vi "KundtsTube.vi"() -> ()   [LabVIEW 2014]
panel:
  in  "Amplitude":dbl
  in  "Stop":bool
  in  "?":enum32{"Sweep", "Single"}(tab)
  in  "Dwell Time":dbl
  in  "Frequency":dbl
  in  "Input 2":T1
  out "RMS":dbl
  out "Waveform Graph":dynamicdata(graph)
  in  "Input":T2
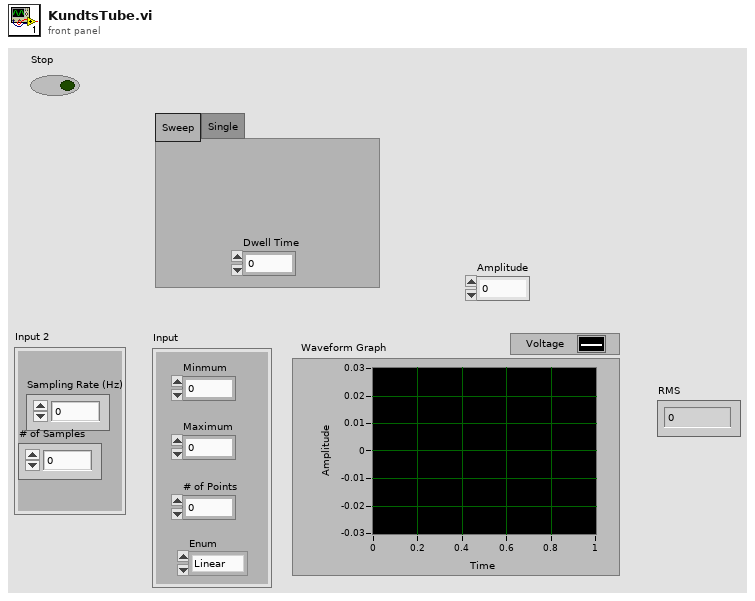
[diagram p1: front panel]
types:
  T1 = cluster{"Sampling Rate (Hz)":dbl, "# of Samples":i64}
  T2 = cluster{"Minmum":i64, "Maximum":i64, "# of Points":i64, "Enum":enum16{"Linear", "Logarithmic", ""}}
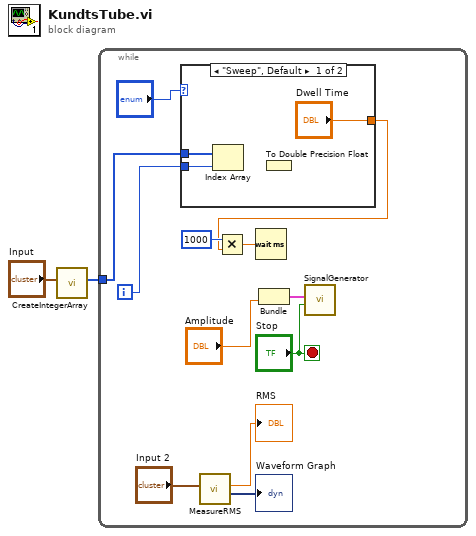
[diagram p0: block diagram]
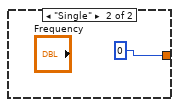
[diagram p2: hidden frame]
diagram:
  n1 = call "CreateIntegerArray.vi"("Input"="Input") -> ("Output Array"=w1:i64[])  [unwired: 10 in]
  n2 = while {
    tunnel: w1 -> [w4]
    i -> [w3]
    stop <- "Stop" stop-if-true
    n3 = case shown="\"Sweep\", Default" "?" {
      tunnel: ["Dwell Time" 0] -> w5
      tunnel: w4 -> [w16 _]
      tunnel: w3 -> [w15 _]
      frame "Sweep", Default {
        n4 = Index Array(array=w16, index=w15) -> ()  [unwired: 1 out]
        n5 = To Double Precision Float() -> ()  [unwired: 1 in, 1 out]
      }
      frame "Single" {
      }
    }
    n6 = call "MeasureRMS.vi"("Input"="Input 2") -> ("Waveform Graph"=→"Waveform Graph":dynamicdata, "RMS"=→"RMS":dbl)  [unwired: 9 in]
    n7 = Multiply(x=1000, y=w5) -> (x*y=w7:dbl)
    n8 = Wait (ms)(milliseconds to wait=w7) -> ()  [unwired: 1 out]
    n9 = Bundle("Amplitude"="Amplitude") -> (w10:cluster{void, "Amplitude":dbl})  [unwired: 2 in]
    n10 = call "SignalGenerator.vi"("Stop"="Stop", "Signal Parameters"=w10) -> ()  [unwired: 10 in]
  }
